vi "niLvFpga_Read32_roboRIO.vi"(0 "session in":u32, 7 "address":u32 format="%.0x", 11 "error in":errorcluster {"code" format="%.0x"}) -> (4 "session out":u32 caption="reference out", 8 "value":u32, 15 "error out":errorcluster {"code" format="%.0x"})   [LabVIEW 2017]
doc: "Performance related peculiarities:\n\n1. Disable the Call Library Function's \"Generate Wrappers\" feature. This feature is displayed when you add the following labview.ini token, and right click on the Call Library Function node:\nextFuncGenNoWrapperEnabled=True\n\n2. For the Call Library function, enable \"Constant\" for parameters >> session.\n\n3. Remove the error case structure around the Call Library Functions. Chaining the errors between multiple Call Library Functions will suffice."
uses:
  <vilib>/rvi/interface/common/niFpgaWaitOnOcc.vi
  NiFpgaLv.dll
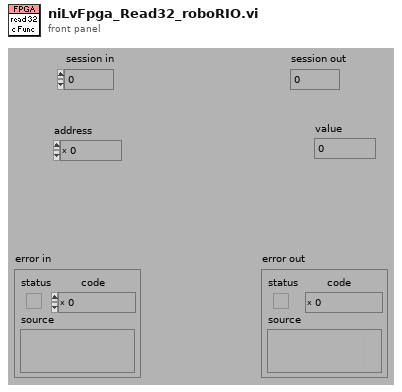
[diagram p1: front panel]
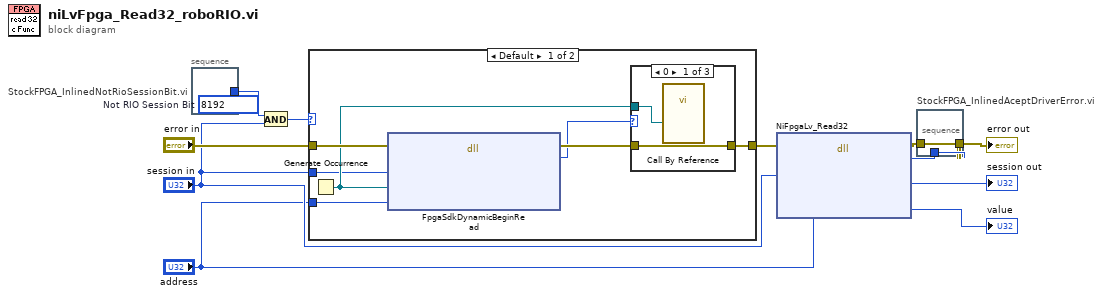
[diagram p0: block diagram]
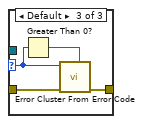
[diagram p4: hidden frame]
diagram:
  n1 = stacked-sequence "StockFPGA_InlinedNotRioSessionBit.vi" {
    tunnel: [w12] -> w5
    frame #0 {
      w12 = u32 8192  # Not RIO Session Bit
    }
  }
  n2 = And(x=w5, y="session in") -> (x .and. y?=w6:u32)
  n3 = case shown="Default" w6 {
    tunnel: "error in" -> [w18 w27]
    tunnel: [w19 w27] -> w3
    tunnel: "session in" -> [w15 _]
    tunnel: "address" -> [w14 _]
    frame Default {
      n4 = Generate Occurrence() -> (w16:refnum<k4>)
      n5 = dll-call lib="LabVIEW" fn="FpgaSdkDynamicBeginRead"(error in=w18, "session"=w15, "occurrence"=w16, "index"=w14) -> (error out=w17:errorcluster, "status"=w13:i32)  [unwired: 5 in, 1 out]
      n6 = case shown="0" w13 {
        selector: w13 -> [_ _ w24]
        tunnel: [w21 w22 w26] -> w19
        tunnel: w16 -> [w20 _ _]
        tunnel: w17 -> [w21 w22 w23]
        frame 0 {
          n7 = call-by-ref "?"("occurrence"=w20) -> ()  [unwired: 16 in, 3 out]
        }
        frame -61167 {
          # "emulation case intentionally ignoring error"
        }
        frame Default {
          n8 = Greater Than 0?(x=w24) -> (x > 0?=w25:bool)
          n9 = call <vilib>:"Error Cluster From Error Code.vi"("is warning? (False)"=w25, "error in (no error)"=w23, "error code (0)"=w24) -> ("error out"=w26:errorcluster)  [unwired: 6 in]
        }
      }
    }
    frame 0 {
    }
  }
  n10 = dll-call lib="NiFpgaLv.*" fn="NiFpgaLv_Read32" label="niLvFpgaRead32"(error in=w3, "session"="session in", "address"="address") -> (error out=w10:errorcluster, "status"=w9:i32, "session"=→"session out":u32, "value"=→"value":u32)  [unwired: 4 in, 1 out]
  n11 = stacked-sequence "StockFPGA_InlinedAceptDriverError.vi" {
    tunnel: w10 -> [w28]
    tunnel: w9 -> [w30]
    tunnel: [w29] -> w8
    frame #0 {
      n12 = case shown="Default" w30 {
        selector: w30 -> [_ w32]
        tunnel: [w31 w34] -> w29
        tunnel: w28 -> [w31 w35]
        frame 0 {
        }
        frame Default {
          n13 = Greater Than 0?(x=w32) -> (x > 0?=w33:bool)
          n14 = call <vilib>:"Error Cluster From Error Code.vi"("is warning? (False)"=w33, "error in (no error)"=w35, "error code (0)"=w32) -> ("error out"=w34:errorcluster)  [unwired: 6 in]
        }
      }
    }
  }
  "error out" <- w8
